vi "BuildHeader.vi"(0 "Tester":string="C Bradshaw", 1 "varnames":string[](array[string]), 2 "Build Sheet File Path":path, 5 "Build Name":string, 7 "raw data filename":string, 9 "Comments on Test":string, 10 "Build Number":string, 11 "Spreadsheet Data":string, 12 "units":string[](array[string]), 13 "steady string":string, 14 "Purpose of Test":string, 15 "Test Request Number":string) -> (4 "Build File Path":path)   [LabVIEW 2017]
panel:
  # "Header"
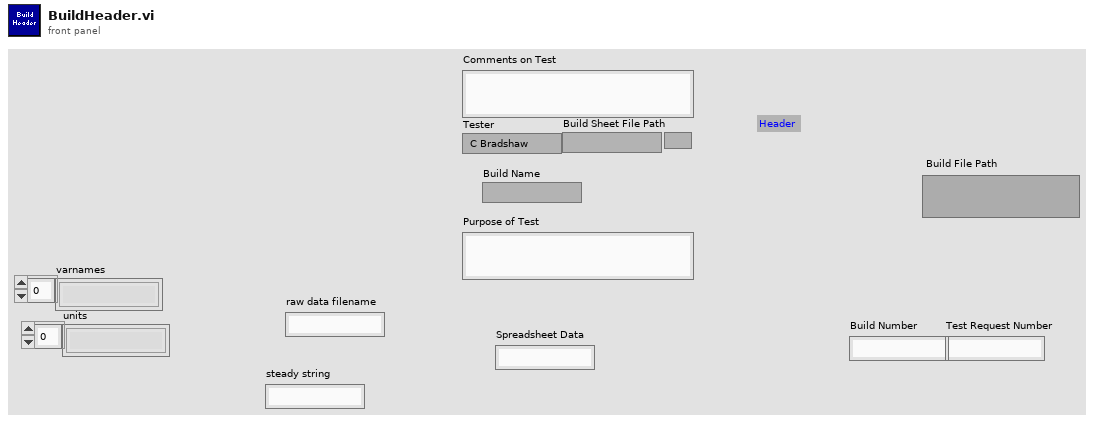
[diagram p1: front panel]
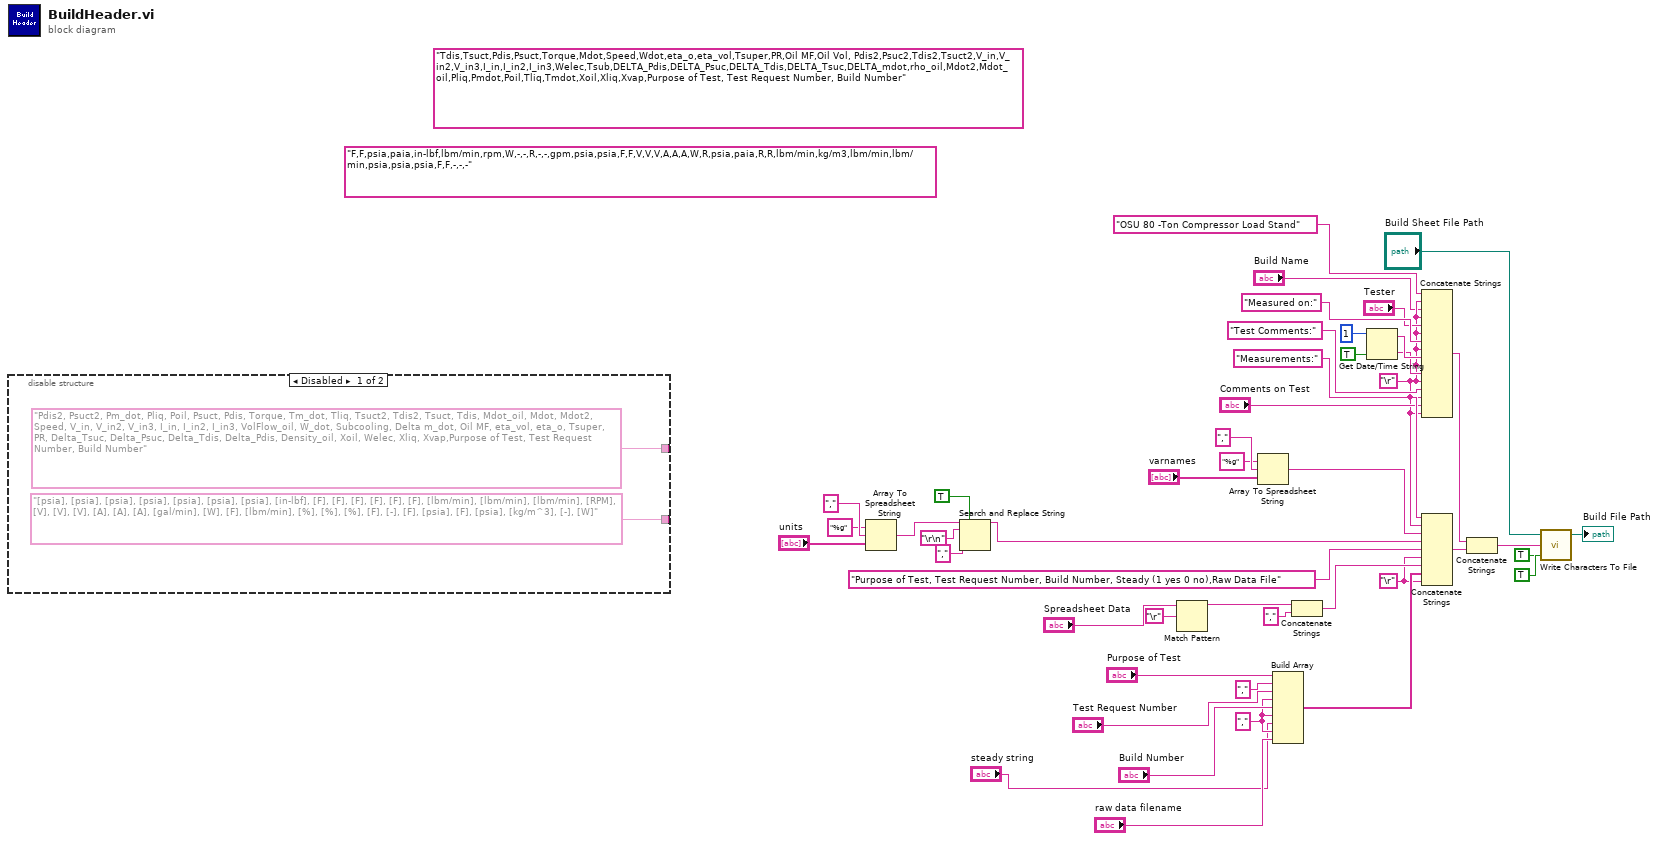
[diagram p0: block diagram]
diagram:
  (unwired) "F,F,psia,paia,in-lbf,lbm/min,rpm,W,-,-,R,-,-,gpm,psia,psia,F,F,V,V,V,A,A,A,W,R,psia,paia,R,R,lbm/min,kg/m3,lbm/min,lbm/min,psia,psia,psia,F,F,-,-,-"
  (unwired) "Tdis,Tsuct,Pdis,Psuct,Torque,Mdot,Speed,Wdot,eta_o,eta_vol,Tsuper,PR,Oil MF,Oil Vol, Pdis2,Psuc2,Tdis2,Tsuct2,V_in,V_in2,V_in3,I_in,I_in2,I_in3,Welec,Tsub,DELTA_Pdis,DELTA_Psuc,DELTA_Tdis,DELTA_Tsuc,DELTA_mdot,rho_oil,Mdot2,Mdot_oil,Pliq,Pmdot,Poil,Tliq,Tmdot,Xoil,Xliq,Xvap,Purpose of Test, Test Request Number, Build Number"
  w2 = "," ("element")
  w8 = "\r"
  w29 = "\r"
  n1 = disable-structure shown="Disabled" {
    disable-tunnel: ["Pdis2, Psuct2, Pm_dot, Pliq, Poil, Psuct, Pdis, Torque, Tm_dot, Tliq, Tsuct2, Tdis2, Tsuct, Tdis, Mdot_oil, Mdot, Mdot2, Speed, V_in, V_in2, V_in3, I_in, I_in2, I_in3, VolFlow_oil, W_dot, Subcooling, Delta m_dot, Oil MF, eta_vol, eta_o, Tsuper, PR, Delta_Tsuc, Delta_Psuc, Delta_Tdis, Delta_Pdis, Density_oil, Xoil, Welec, Xliq, Xvap,Purpose of Test, Test Request Number, Build Number" _] -> _
    disable-tunnel: ["[psia], [psia], [psia], [psia], [psia], [psia], [psia], [in-lbf], [F], [F], [F], [F], [F], [F], [lbm/min], [lbm/min], [lbm/min], [RPM], [V], [V], [V], [A], [A], [A], [gal/min], [W], [F], [lbm/min], [%], [%], [%], [F], [-], [F], [psia], [F], [psia], [kg/m^3], [-], [W]" _] -> _
    frame Disabled {
    }
    frame Enabled {
    }
  }
  n2 = Array To Spreadsheet String(delimiter (Tab)=",", array="units", 3:"%g" ("format string")) -> (spreadsheet string=w6:string)
  n3 = Search and Replace String(replace all?=TRUE ("replace all? (F)"), input string=w6, search string="\r\n", replace string="," ("replace string (\"\")")) -> (result string=w4:string)  [unwired: 4 in, 3 out]
  n4 = Match Pattern(string="Spreadsheet Data", regular expression="\r") -> (before substring=w23:string)  [unwired: 1 in, 3 out]
  n5 = Array To Spreadsheet String(delimiter (Tab)=",", array="varnames", 3:"%g" ("format string")) -> (spreadsheet string=w10:string)
  n6 = Build Array("Purpose of Test", "," ("element"), "Test Request Number", w2, "Build Number", w2, "steady string", w2, "raw data filename") -> (w18:string[])
  n7 = Concatenate Strings(w23, "," ("string")) -> (w24:string)
  n8 = Get Date/Time String(date format (0)=1, want seconds? (F)=TRUE) -> (date string=w43:string, time string=w42:string)  [unwired: 1 in]
  n9 = Concatenate Strings("OSU 80 -Ton Compressor Load Stand", w29, "Build Name", w29, "Tester", w29, "Measured on:", w29, w43, w29, w42, w29, "Test Comments:", w29, "Comments on Test", w29) -> (w39:string)
  n10 = Concatenate Strings("Measurements:", w29, w10, w4, "Purpose of Test, Test Request Number, Build Number, Steady (1 yes 0 no),Raw Data File", w8, w24, w18, w8) -> (w38:string)
  n11 = Concatenate Strings(w39, w38) -> (w37:string)
  n12 = call <vilib>:"Write Characters To File.vi"("convert eol? (no:F)"=TRUE, "append to file? (new file:F)"=TRUE, "character string"=w37, "file path (dialog if empty)"="Build Sheet File Path") -> ("new file path (Not A Path if cancelled)"=→"Build File Path":path)  [unwired: 1 in]
